vi "Store Step Result.vi"(7 "Vacuum?":bool=TRUE, 10 "Step Result":T2, 11 "Test Results In":T1) -> (3 "Test Results Out":T1)   [LabVIEW 2015]
uses:
  Controls/Step Result.ctl
  Controls/Test Results.ctl
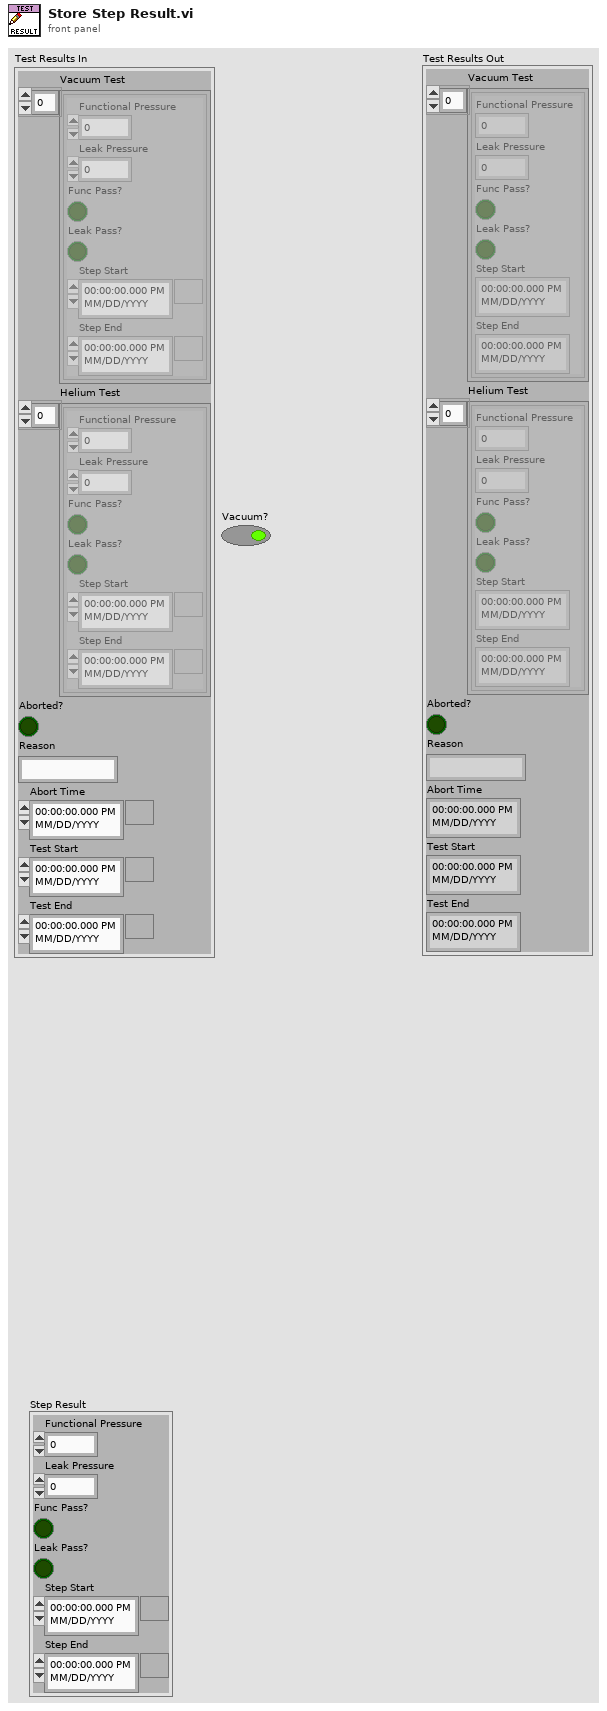
[diagram p1: front panel]
types:
  T1 = typedef "Test Results.ctl" = cluster{"Vacuum Test":T2[], "Helium Test":T2[], "Aborted?":bool, "Reason":string, "Abort Time":timestamp, "Test Start":timestamp, "Test End":timestamp}
  T2 = typedef "Step Result.ctl" = cluster{"Functional Pressure":dbl, "Leak Pressure":dbl, "Func Pass?":bool, "Leak Pass?":bool, "Step Start":timestamp, "Step End":timestamp}
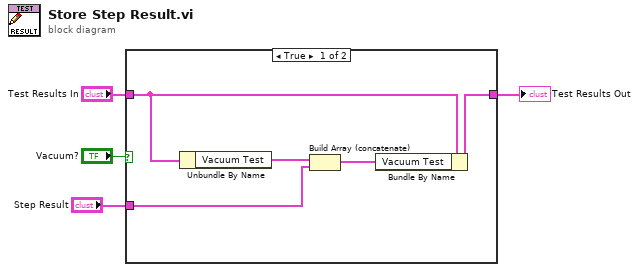
[diagram p0: block diagram]
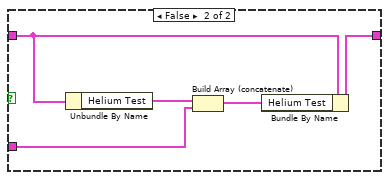
[diagram p2: hidden frame]
diagram:
  n1 = case shown="True" "Vacuum?" {
    tunnel: "Step Result" -> [w8 w13]
    tunnel: "Test Results In" -> [w6 w11]
    tunnel: [w5 w10] -> w2
    frame True {
      n2 = Unbundle By Name(w6) -> ("Vacuum Test"=w7:T2[])
      n3 = Build Array (concatenate)(w7, w8) -> (w9:T2[])
      n4 = Bundle By Name(cluster=w6, "Vacuum Test"=w9) -> (w5:T1)
    }
    frame False {
      n5 = Unbundle By Name(w11) -> ("Helium Test"=w12:T2[])
      n6 = Build Array (concatenate)(w12, w13) -> (w14:T2[])
      n7 = Bundle By Name(cluster=w11, "Helium Test"=w14) -> (w10:T1)
    }
  }
  "Test Results Out" <- w2
